vi "User Event Handler.vi"(7 "User Event Action":T1, 8 "error in (no error)":errorcluster) -> (0 "error out":errorcluster, 3 "User Event - Stop":refnum<user-event>)   [LabVIEW 2020, in "User Event - Stop.lvlib"]
doc: "Main User Event handler."
uses:
  User Event - Stop.lvlib
  Controls/User event Actions.ctl
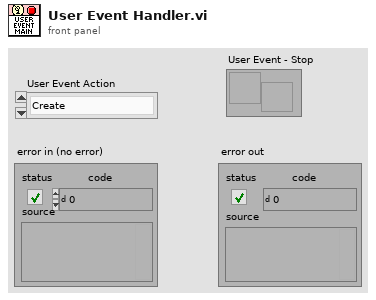
[diagram p1: front panel]
types:
  T1 = typedef "User Event - Stop.lvlib/User event Actions.ctl" = enum16{"Create", "Get Reference", "Fire Stop Event", "Destroy"}
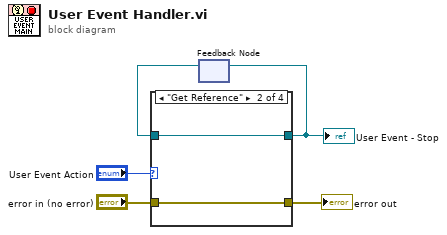
[diagram p0: block diagram]
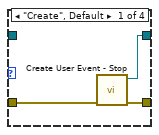
[diagram p2: hidden frame]
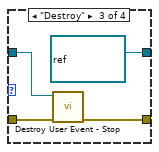
[diagram p3: hidden frame]
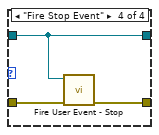
[diagram p4: hidden frame]
diagram:
  n1 = feedback #1() -> (w1:refnum<user-event>)  [unwired: 1 in]
  n2 = case shown="\"Get Reference\"" "User Event Action" {
    tunnel: "error in (no error)" -> [w8 w9 w13 w17]
    tunnel: [w7 w9 w14 w16] -> w3
    tunnel: [w6 w10 refnum<user-event> refnum ("User Event - Stop") w15] -> w2
    tunnel: w1 -> [_ w10 w12 w15]
    frame "Create", Default {
      n3 = call "Create User Event - Stop.vi"("error in (no error)"=w8) -> ("error out"=w7:errorcluster, "User Event - Stop"=w6:refnum<user-event>)  [unwired: 9 in]
    }
    frame "Get Reference" {
    }
    frame "Destroy" {
      n4 = call "Destroy User Event - Stop.vi"("error in (no error)"=w13, "User Event - Stop"=w12) -> ("error out"=w14:errorcluster)  [unwired: 9 in]
    }
    frame "Fire Stop Event" {
      n5 = call "Fire User Event - Stop.vi"("error in (no error)"=w17, "User Event - Stop"=w15) -> ("error out"=w16:errorcluster)  [unwired: 9 in]
    }
  }
  "error out" <- w3
  "User Event - Stop" <- w2
  n6 = feedback-in #1(w2) -> ()
